vi "Meter Detection RT Driver VI.vi"(6 "Device Clock":string, 9 "Device Inputs FIFO":refnum<k33>, 10 "Device Outputs FIFO":refnum<k33>, 11 "Device Reference":T1 format="%.0x") -> ()   [LabVIEW 2011, in "Meter Detection Custom Device.lvlib"]
uses:
  Meter Detection Custom Device.lvlib
  <vilib>/NI Veristand/Custom Device API/Custom Device Item Ref.ctl
  <vilib>/NI Veristand/Custom Device API/Message Response (String).ctl
  <vilib>/NI Veristand/Custom Device API/Message Response (Byte Array).ctl
  <vilib>/NI Veristand/Custom Device Tools/Custom Device Utility Library/Custom Device Utility Library.lvlib
  <vilib>/NI Veristand/Custom Device API/Custom Device API.lvlib
  <vilib>/vision/driver/NI_Vision_Acquisition_Software.lvlib
  <vilib>/vision/NI_Vision_Development_Module.lvlib
panel:
  in  "Initialization Status Notifier":refnum<notifier>
  in  "Status Notifier":refnum<notifier>
  # "Custom Device Template\nv1.0"
  # "Use this template as a starting point for creating a custom device code module. The input controls shown here are specially named controls that the system will use to provide the device loop with data. The controls are not required for the device loop to run. For instance, if the device doesn't produce any output data, then you don't need the Device Outputs FIFO control. If you do use these controls, however, they need to have these exact names to be functional."
  # "The optional status notifier element is used to notify the RT engine of the last state of the custom device, and to indicate the device has completed execution. If this control is not used, a default No Error value is returned to the system when the device finishes execution.\n\nNote: This error state is not checked until the system shuts down. Use an output status channel to send more immediate status values to the system."
  # "This optional input can be used to send the VeriStand Engine the final status of the custom device initalization process. If this control exists on the custom device front panel, the VeriStand Engine will wait for a status update before starting up. If the custom device reports an error, that will abort the execution of the current configuration in the VeriStand Engine.\n\nThis control can be deleted if the custom device does not need to send the initialization status update."
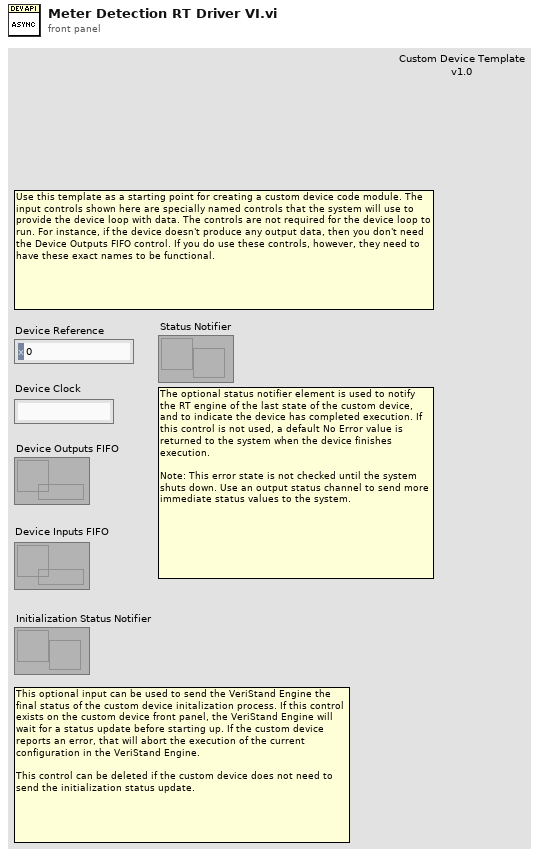
[diagram p1: front panel]
types:
  T1 = typedef "Custom Device API.lvlib/Custom Device Item Ref.ctl" = u64
  T2 = typedef "Custom Device API.lvlib/Custom Device Engine Event Ref.ctl" = refnum<event-registration>
  T3 = typedef "IMAQdx.ctl" = refnum<k21>
  T4 = typedef "IMAQ Image.ctl" = refnum<image>
  T5 = typedef "Custom Device API.lvlib/Message Response (String).ctl" = cluster{"Response":string, "Error":errorcluster}
  T6 = typedef "Custom Device API.lvlib/Message Response (Byte Array).ctl" = cluster{"Response":u8[], "Error":errorcluster}
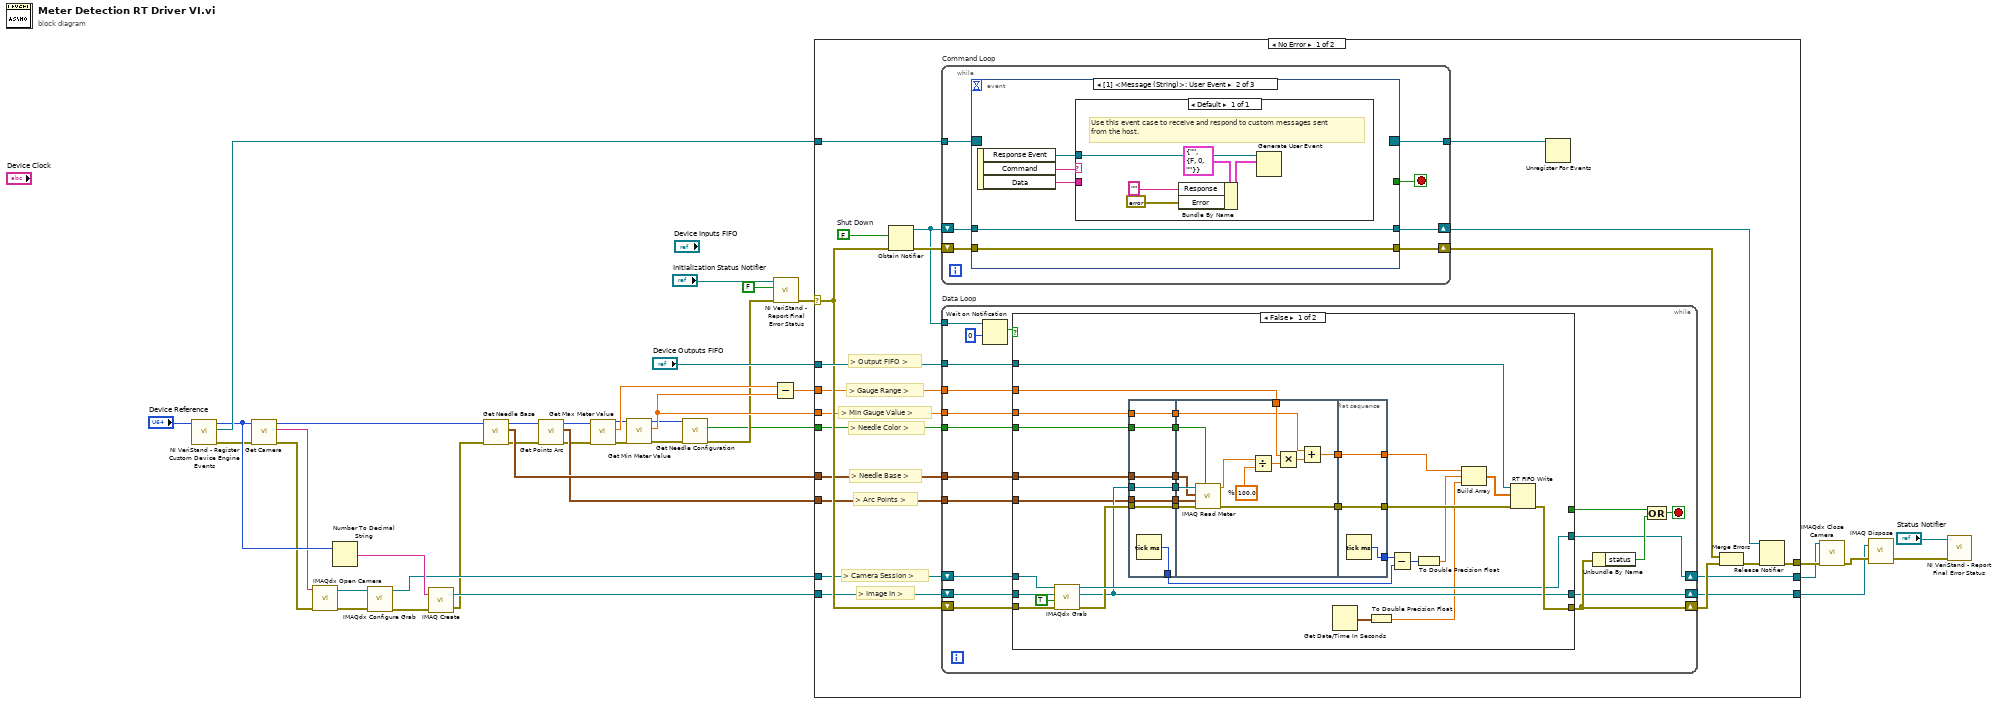
[diagram p0: block diagram]
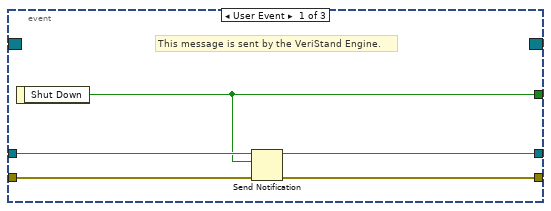
[diagram p2: hidden frame]
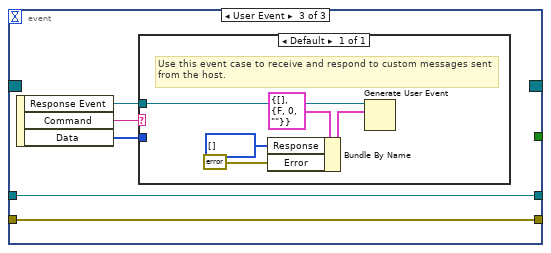
[diagram p3: hidden frame]
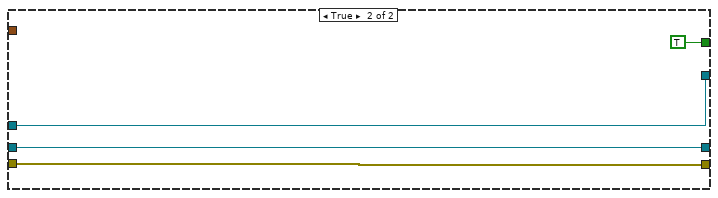
[diagram p4: hidden frame]
diagram:
  n1 = call <vilib>:"NI VeriStand - Register Custom Device Engine Events.vi"("Device Ref in"="Device Reference") -> ("error out"=w19:errorcluster, "Custom Device Engine Event Ref"=w36:T2, "Device Ref out"=w20:T1)  [unwired: 8 in]
  n2 = call "Get Camera.vi"("error in (no error)"=w19, "Item Ref out in"=w20) -> ("error out"=w18:errorcluster, "Camera"=w17:string, "Item Ref out out"=w15:T1)  [unwired: 7 in]
  n3 = call <vilib>:"IMAQdx Open Camera.vi"("error in"=w18, "Session In"=w17) -> ("error out"=w32:errorcluster, "Session Out"=w31:T3)  [unwired: 8 in]
  n4 = Number To Decimal String(number=w20) -> (decimal integer string=w29:string)  [unwired: 1 in]
  n5 = call <vilib>:"IMAQdx Configure Grab.vi"("error in"=w32, "Session In"=w31) -> ("error out"=w30:errorcluster, "Session Out"=w28:T3)  [unwired: 8 in]
  n6 = call "IMAQ Create"("Image Name"=w29, "error in (no error)"=w30) -> ("New Image"=w27:T4, "error out"=w16:errorcluster)  [unwired: 3 in]
  n7 = call "Get Needle Base.vi"("error in (no error)"=w16, "Item Ref in"=w15) -> ("error out"=w13:errorcluster, "Needle Base"=w14:cluster{"X":sgl, "Y":sgl}, "Item Ref out"=w12:T1)  [unwired: 7 in]
  n8 = call "Get Points Arc.vi"("error in (no error)"=w13, "Item Ref in"=w12) -> ("error out"=w8:errorcluster, "Points Arc"=w11:cluster{"X":sgl, "Y":sgl}[], "Item Ref out"=w9:T1)  [unwired: 7 in]
  n9 = call "Get Max Meter Value.vi"("error in (no error)"=w8, "Item Ref in"=w9) -> ("error out"=w7:errorcluster, "Max Gauge Value"=w10:dbl, "Item Ref out"=w6:T1)  [unwired: 7 in]
  n10 = call "Get Min Meter Value.vi"("error in (no error)"=w7, "Item Ref in"=w6) -> ("error out"=w4:errorcluster, "Min Gauge Value"=w5:dbl, "Item Ref out"=w3:T1)  [unwired: 7 in]
  n11 = call "Get Needle Configuration.vi"("error in (no error)"=w4, "Item Ref in"=w3) -> ("error out"=w2:errorcluster, "Needle Configuration out"=w1:bool)  [unwired: 7 in, 1 out]
  n12 = Subtract(x=w10, y=w5) -> (x-y=w21:dbl)
  n13 = call <vilib>:"NI VeriStand - Report Final Error Status.vi"("error in (no error)"=w2, "Filter FIFO Errors (T)"=FALSE, "Status Notifier"="Initialization Status Notifier") -> ("error out"=w34:errorcluster)  [unwired: 8 out]
  n14 = case shown="No Error" w34 {
    selector: w34 -> [w51 w171]
    tunnel: "Device Outputs FIFO" -> [w59 _]
    tunnel: w36 -> [w58 _]
    tunnel: [w56 w171] -> w26
    tunnel: w28 -> [w48 w170]
    tunnel: w27 -> [w47 w169]
    tunnel: [w46 w170] -> w25
    tunnel: [w45 w169] -> w22
    tunnel: w5 -> [w44 _]
    tunnel: w21 -> [w41 _]
    tunnel: w11 -> [w42 _]
    tunnel: w14 -> [w43 _]
    tunnel: w1 -> [w40 _]
    frame No Error {
      w57 = FALSE  # Shut Down
      # "> Needle Color >"
      # "> Image In >"
      # "> Camera Session >"
      # "> Arc Points >"
      # "> Needle Base >"
      # "> Output FIFO >"
      # "> Min Gauge Value >"
      # "> Gauge Range >"
      n15 = Obtain Notifier(notification data type=w57, error in (no error)=w51) -> (notifier out=w54:refnum<notifier>, error out=w60:errorcluster)  [unwired: 2 in, 1 out]
      n16 = while "Command Loop" {
        tunnel: w58 -> [w67]
        tunnel: [w66] -> w55
        shift-right: [w63] -> w53
        shift-left: w54 -> [w64]
        shift-right: [w61] -> w49
        shift-left: w60 -> [w62]
        stop <- w65 stop-if-true
        n17 = event shown="[1] <Message (String)>: User Event" {
          selector: w67 -> [_ _ _]
          dyn-events: [_ _ _] -> w66
          timeout: _ -> [_ _ _]
          tunnel: [w70 _ _] -> w65
          tunnel: w64 -> [w71 w75 w85]
          tunnel: [w72 w75 w85] -> w63
          tunnel: w62 -> [w69 w73 w83]
          tunnel: [w68 w73 w83] -> w61
          event User Event {
            # "This message is sent by the VeriStand Engine."
            n18 = event-data() -> ("Shut Down"=w70:bool)  [unwired: 1 in]
            n19 = Send Notification(notification=w70, notifier=w71, error in (no error)=w69) -> (notifier out=w72:refnum<notifier>, error out=w68:errorcluster)
          }
          event User Event {
            n20 = event-data() -> ("Response Event"=w74:refnum<user-event>, "Command"=w77:string, "Data"=w76:string)  [unwired: 1 in]
            n21 = case shown="Default" w77 {
              tunnel: w76 -> [_]
              tunnel: w74 -> [w82]
              frame Default {
                # "Use this event case to receive and respond to custom messages sent from the host."
                n22 = Bundle By Name(cluster=T5 {"Response"="", "Error"={"status"=FALSE, "code"=0, "source"=""}} ("event data"), "Response"="", "Error"=errorcluster {"status"=FALSE, "code"=0, "source"=""}) -> (w80:T5)
                n23 = Generate User Event(user event=w82, event data cluster=w80) -> ()  [unwired: 1 in, 2 out]
              }
            }
          }
          event User Event {
            n24 = event-data() -> ("Response Event"=w84:refnum<user-event>, "Command"=w87:string, "Data"=w86:u8[])  [unwired: 1 in]
            n25 = case shown="Default" w87 {
              tunnel: w86 -> [_]
              tunnel: w84 -> [w92]
              frame Default {
                # "Use this event case to receive and respond to custom messages sent from the host."
                n26 = Bundle By Name(cluster=T6 {"Response"=[], "Error"={"status"=FALSE, "code"=0, "source"=""}} ("event data"), "Response"=u8[] [], "Error"=errorcluster {"status"=FALSE, "code"=0, "source"=""}) -> (w89:T6)
                n27 = Generate User Event(user event=w92, event data cluster=w89) -> ()  [unwired: 1 in, 2 out]
              }
            }
          }
        }
      }
      n28 = while "Data Loop" {
        shift-right: [w107] -> w52
        shift-left: w51 -> [w110]
        tunnel: w59 -> [w109]
        tunnel: w54 -> [w106]
        shift-right: [w99] -> w46
        shift-left: w48 -> [w101]
        shift-right: [w98] -> w45
        shift-left: w47 -> [w100]
        tunnel: w44 -> [w94]
        tunnel: w43 -> [w97]
        tunnel: w42 -> [w96]
        tunnel: w41 -> [w95]
        tunnel: w40 -> [w93]
        stop <- w102 stop-if-true
        n29 = Wait on Notification(notifier=w106, timeout in ms (-1)=0) -> (notification=w105:bool)  [unwired: 2 in, 3 out]
        n30 = case shown="False" w105 {
          tunnel: w110 -> [w139 w168]
          tunnel: w109 -> [w141 _]
          tunnel: [w140 w168] -> w107
          tunnel: [_ TRUE] -> w103
          tunnel: w101 -> [w138 w166]
          tunnel: w100 -> [w137 w165]
          tunnel: [w136 w166] -> w99
          tunnel: [w133 w165] -> w98
          tunnel: w97 -> [w132 _]
          tunnel: w96 -> [w131 _]
          tunnel: w95 -> [w130 _]
          tunnel: w94 -> [w129 _]
          tunnel: w93 -> [w112 _]
          frame False {
            n31 = call <vilib>:"IMAQdx Grab.vi"("error in"=w139, "Wait for Next Buffer? (Yes)"=TRUE, "Image In"=w137, "Session In"=w138) -> ("error out"=w135:errorcluster, "Image Out"=w133:T4, "Session Out"=w136:T3)  [unwired: 4 in, 1 out]
            n32 = flat-sequence {
              tunnel: w129 -> [w144]
              tunnel: w131 -> [w145]
              tunnel: w132 -> [w146]
              tunnel: w133 -> [w147]
              tunnel: w135 -> [w148]
              tunnel: [w148] -> w128
              tunnel: [w147] -> w127
              tunnel: [w146] -> w126
              tunnel: [w145] -> w125
              tunnel: [w144] -> w124
              tunnel: [w143] -> w121
              tunnel: w112 -> [w142]
              tunnel: [w142] -> w111
              tunnel: w130 -> [w153]
              tunnel: w128 -> [w161]
              tunnel: w127 -> [w159]
              tunnel: w126 -> [w158]
              tunnel: w125 -> [w157]
              tunnel: w124 -> [w151]
              tunnel: [w160] -> w123
              tunnel: [w150] -> w115
              tunnel: w111 -> [w149]
              tunnel: [w164] -> w134
              tunnel: w123 -> [w164]
              tunnel: [w163] -> w122
              tunnel: w115 -> [w162]
              tunnel: [w162] -> w114
              frame #0 {
                n33 = Tick Count (ms)() -> (millisecond timer value=w143:u32)
              }
              frame #1 {
                w155 = 100.0  # %
                n34 = call "IMAQ Read Meter"("Needle color"=w149, "error in (no error)"=w161, "Arc Points"=w157, "Needle Base"=w158, "Image"=w159) -> ("error out"=w160:errorcluster, "Percentage of scale"=w156:dbl)  [unwired: 4 in, 1 out]
                n35 = Divide(x=w156, y=w155) -> (x/y=w154:dbl)
                n36 = Multiply(x=w153, y=w154) -> (x*y=w152:dbl)
                n37 = Add(x=w151, y=w152) -> (x+y=w150:dbl)
              }
              frame #2 {
                n38 = Tick Count (ms)() -> (millisecond timer value=w163:u32)
              }
            }
            n39 = Get Date/Time In Seconds() -> (seconds since 1Jan1904=w117:timestamp)
            n40 = To Double Precision Float(number=w117) -> (double precision float=w116:dbl)
            n41 = Subtract(x=w122, y=w121) -> (x-y=w119:u32)
            n42 = To Double Precision Float(number=w119) -> (double precision float=w118:dbl)
            n43 = Build Array(w114, w118, w116) -> (w120:dbl[])
            n44 = RT FIFO Write(0:w141, 1:w120, 3:w134) -> (11:w140:errorcluster)  [unwired: 1 in, 4 out]
          }
          frame True {
          }
        }
        n45 = Unbundle By Name(w107) -> ("status"=w104:bool)
        n46 = Compound Arithmetic op=OR(w103, w104) -> (w102:bool)
      }
      n47 = Unregister For Events(event registration refnum=w55) -> ()  [unwired: 1 in, 1 out]
      n48 = Merge Errors(w49, w52) -> (w50:errorcluster)
      n49 = Release Notifier(notifier=w53, error in (no error)=w50) -> (error out=w56:errorcluster)  [unwired: 1 in, 2 out]
    }
    frame Error {
    }
  }
  n50 = call <vilib>:"IMAQdx Close Camera.vi"("error in"=w26, "Session In"=w25) -> ("error out"=w24:errorcluster)  [unwired: 9 in]
  n51 = call "IMAQ Dispose"("Image"=w22, "error in (no error)"=w24) -> ("error out"=w23:errorcluster)  [unwired: 4 in]
  n52 = call <vilib>:"NI VeriStand - Report Final Error Status.vi"("error in (no error)"=w23, "Status Notifier"="Status Notifier") -> ()  [unwired: 1 in, 9 out]
